vi "Read ADU Packet.vi"(8 "error in":errorcluster, 10 "protocol layer":refnum<class "Network Protocol.lvclass">, 11 "RTU transmission data unit in":refnum<class "RTU Data Unit.lvclass">) -> (0 "error out":errorcluster, 1 "modbus data unit":refnum<class "Modbus Data Unit (PDU).lvclass">, 2 "protocol layer out":refnum<class "Network Protocol.lvclass">, 3 "RTU transmission data unit out":refnum<class "RTU Data Unit.lvclass">, 5 "PDU Valid?":bool)   [LabVIEW 2020, in "SubVIs.lvlib" / "RTU Data Unit.lvclass"]
doc: "This uses the protocol layer to read a modbus packet off of the bus, wrapped in the RTU transmission data unit."
uses:
  <vilib>/Modbus/subvis/Transmission Data Unit (ADU)/RTU Data Unit/RTU Data Unit.lvclass
  C:/builds/penguin/iak/lvdsc/trunk/20.0/lv/vi.lib/Modbus/subvis/Transmission Data Unit (ADU)/Transmission Data Unit/Transmission Data Unit.lvclass
  C:/builds/penguin/iak/lvdsc/trunk/20.0/lv/vi.lib/Modbus/subvis/Transmission Data Unit (ADU)/Serial Data Unit/Serial Data Unit.lvclass
  <vilib>/Modbus/subvis/Modbus Data Unit (PDU)/Modbus Data Unit (PDU).lvclass
  <vilib>/Modbus/subvis/Protocol/Interfaces/Network Protocol/Network Protocol.lvclass
  <vilib>/Modbus/subvis/Protocol/Serial/Serial Slave/Serial Slave.lvclass
  <vilib>/Modbus/subvis/Protocol/Serial/Serial Master/Serial Master.lvclass
  <vilib>/Modbus/subvis/Protocol/Serial/Serial Master/Serial Master.lvclass/Serial Master.ctl
  <vilib>/Modbus/subvis/Protocol/Serial/Serial Slave/Serial Slave.lvclass/Serial Slave.ctl
  <vilib>/Modbus/subvis/Transmission Data Unit (ADU)/Transmission Data Unit/Transmission Data Unit.lvclass/Transmission Data Unit.ctl
  <vilib>/Modbus/subvis/Transmission Data Unit (ADU)/Serial Data Unit/Serial Data Unit.lvclass/Serial Data Unit.ctl
  <vilib>/Modbus/subvis/Modbus Data Unit (PDU)/Modbus Data Unit (PDU).lvclass/Modbus Data Unit (PDU).ctl
  <vilib>/ErrorRing/Error Ring.xnode
  <vilib>/Modbus/subvis/Transmission Data Unit (ADU)/Serial Data Unit/Serial Data Unit.lvclass
  <vilib>/Modbus/subvis/Transmission Data Unit (ADU)/Transmission Data Unit/Transmission Data Unit.lvclass
  <vilib>/Modbus/subvis/Protocol/Serial/Serial Shared Components/Serial Shared Components.lvlib
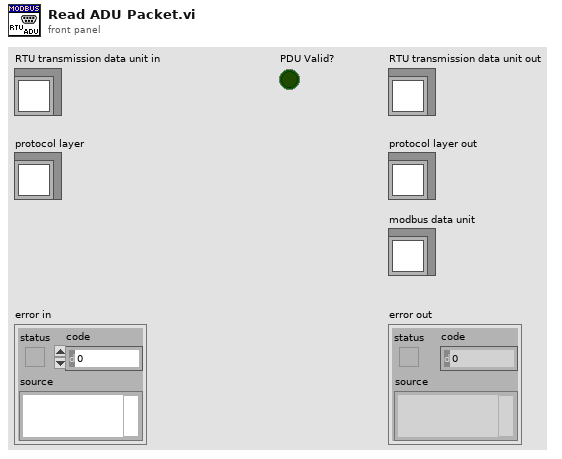
[diagram p1: front panel]
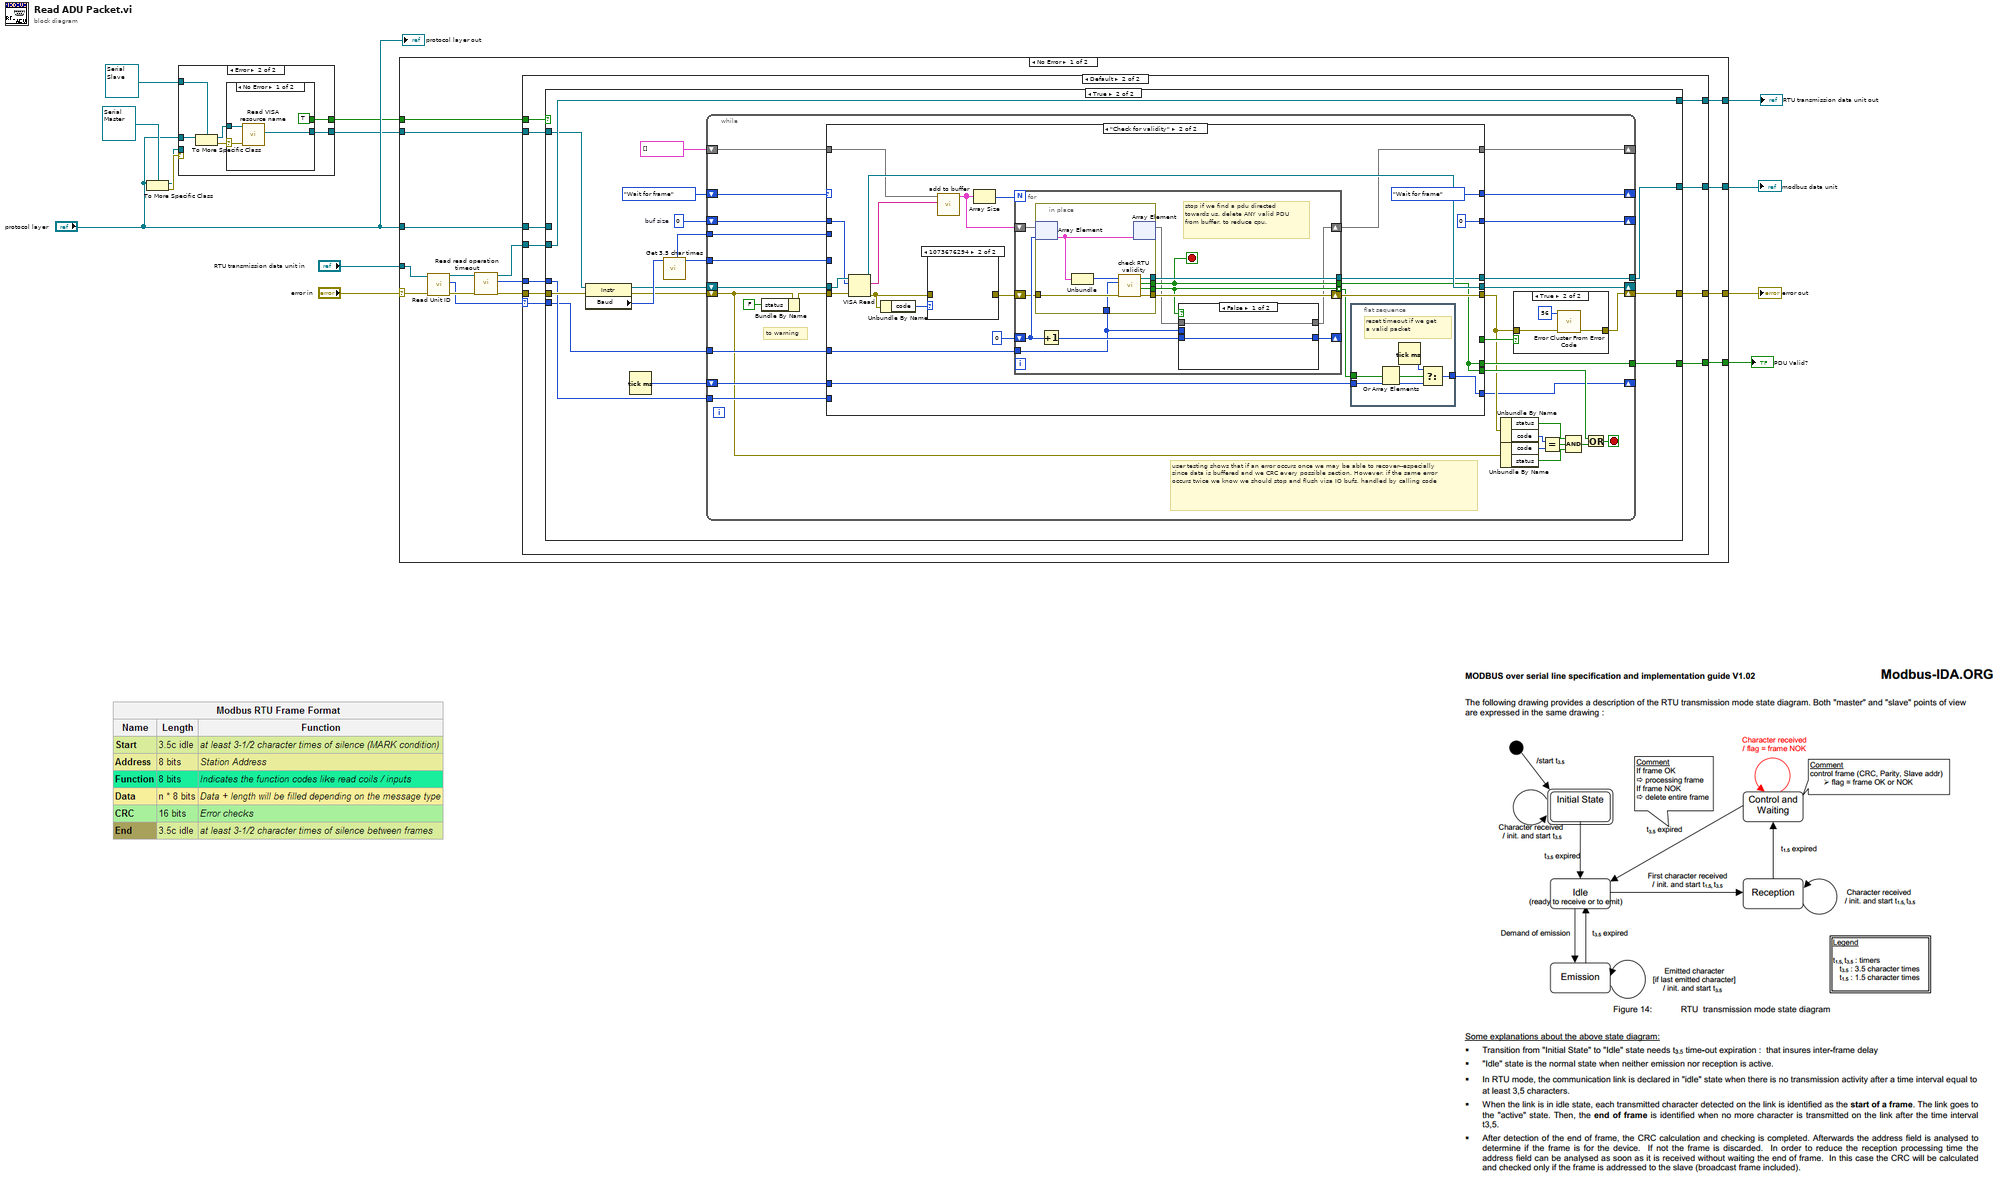
[diagram p0: block diagram]
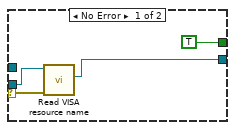
[diagram p2: hidden frame]
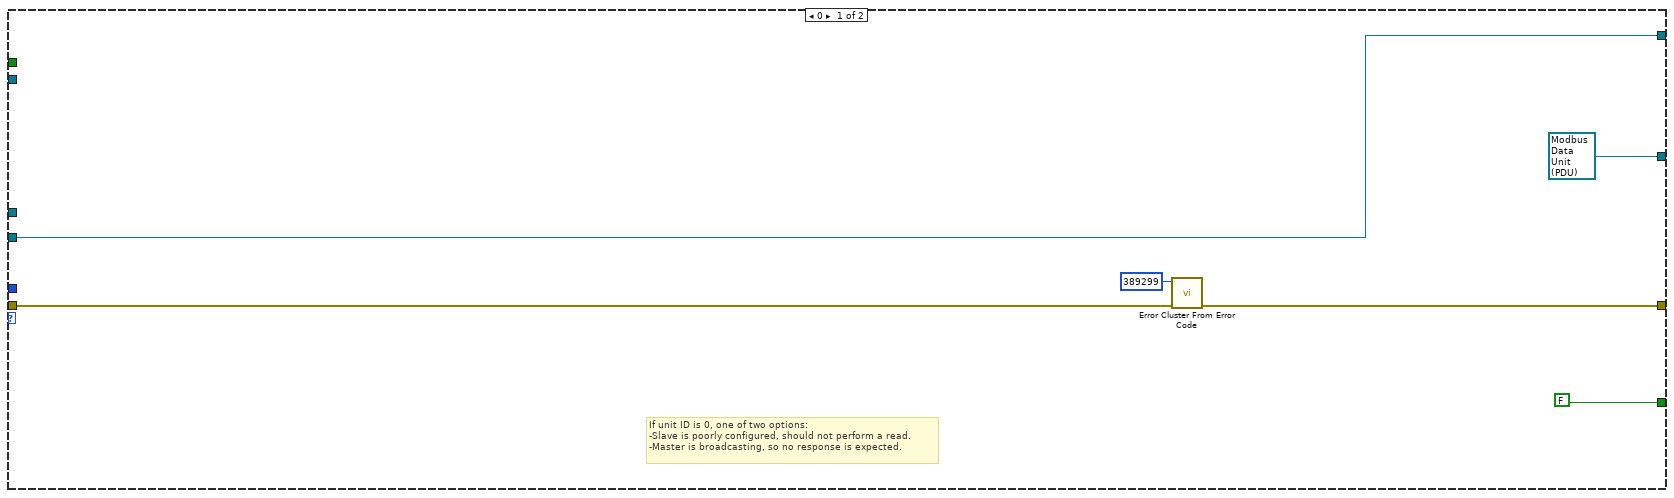
[diagram p4: hidden frame]
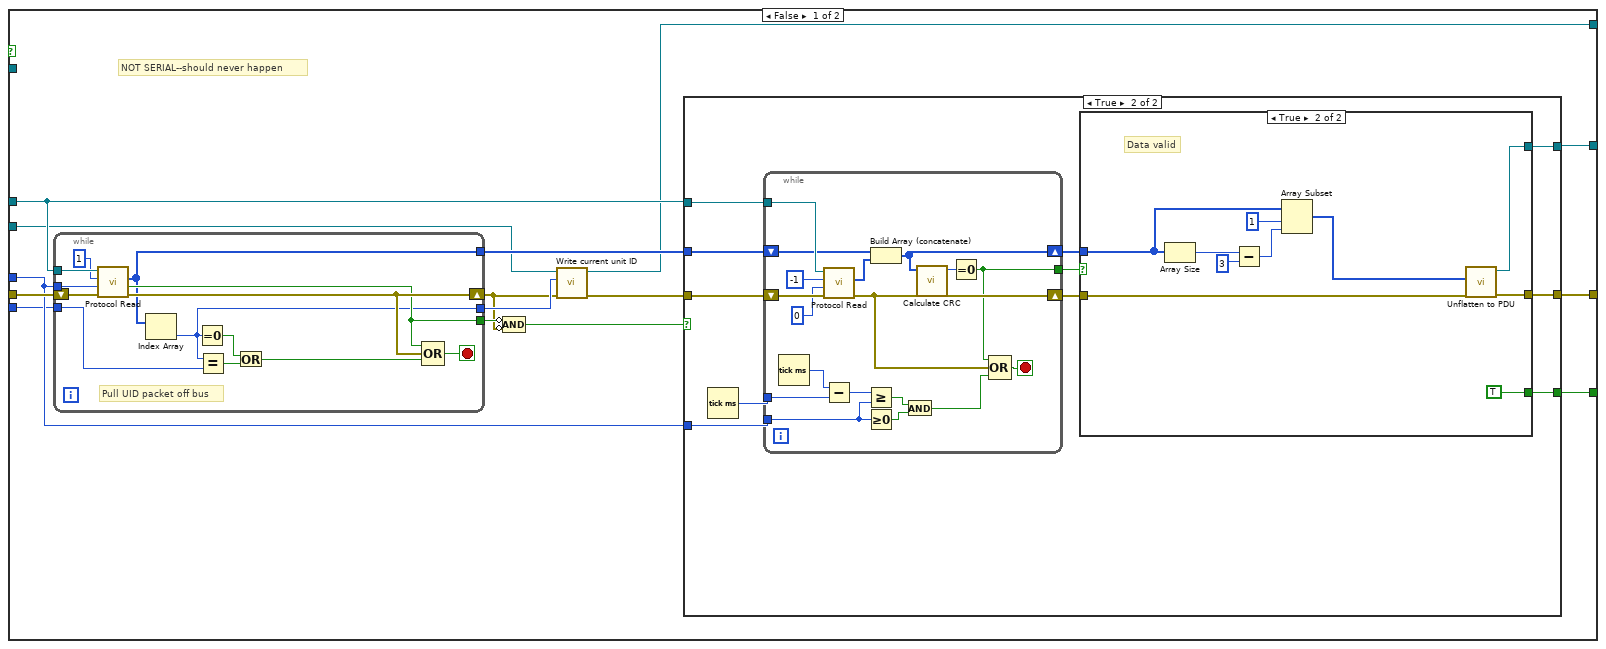
[diagram p5: hidden frame]
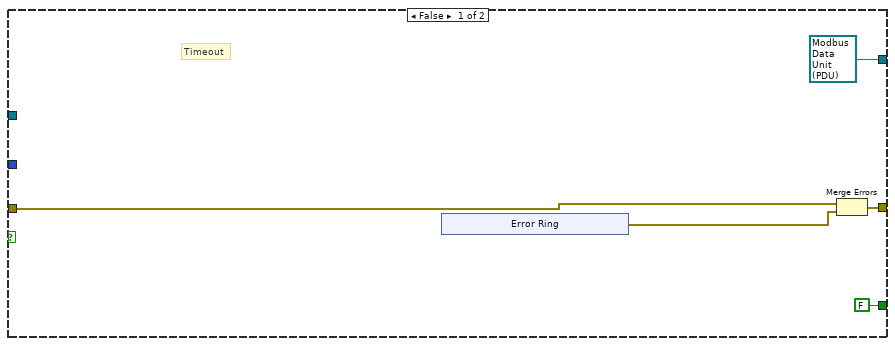
[diagram p6: hidden frame]
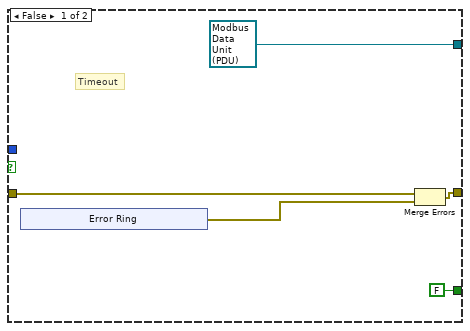
[diagram p7: hidden frame]
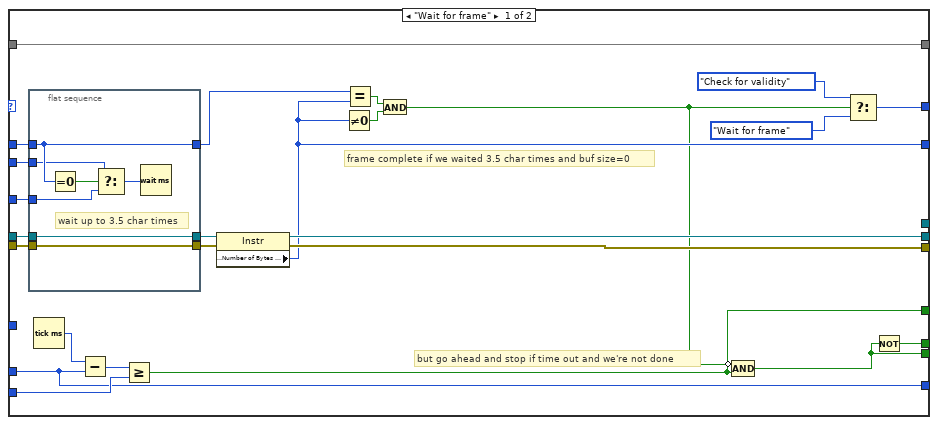
[diagram p9: hidden frame]
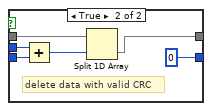
[diagram p11: hidden frame]
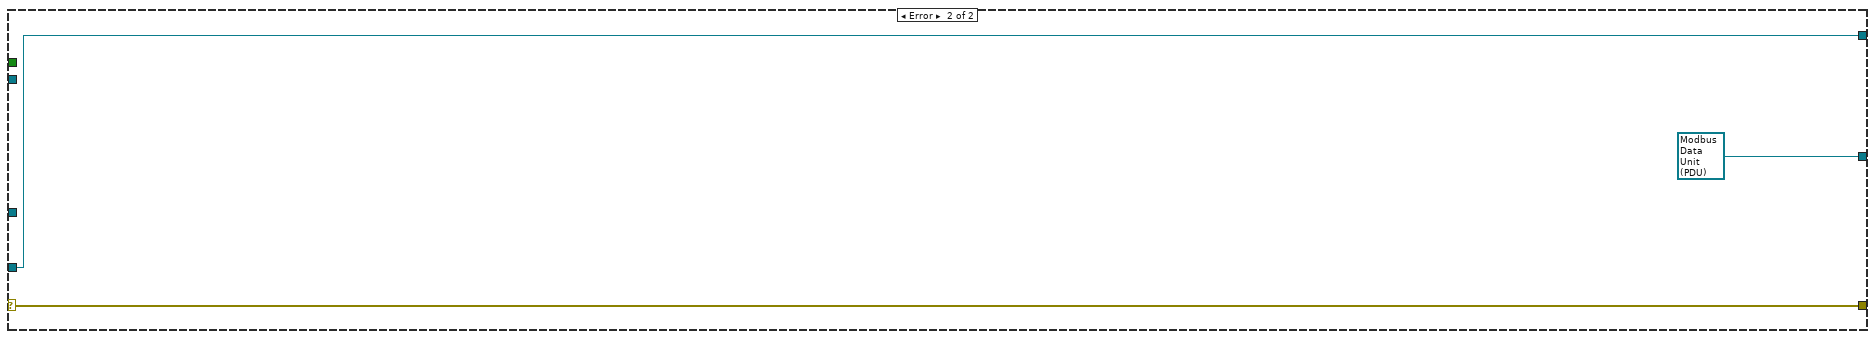
[diagram p12: hidden frame]
diagram:
  n1 = To More Specific Class(target class=refnum<class "Serial Master.lvclass"> refnum ("Serial Master"), reference="protocol layer") -> (specific class reference=w2:refnum<class "Serial Master.lvclass">, error out=w6:errorcluster)  [unwired: 1 in]
  n2 = case shown="Error" w6 {
    selector: w6 -> [w16 _]
    tunnel: "protocol layer" -> [_ w23]
    tunnel: [TRUE w21] -> w4
    tunnel: refnum<class "Serial Slave.lvclass"> refnum ("Serial Slave") -> [_ w20]
    tunnel: [w14 w18] -> w1
    tunnel: w2 -> [w15 _]
    frame No Error {
      n3 = call <vilib>:"Read VISA resource name.vi"("error in (no error)"=w16, "serial master in"=w15) -> ("VISA resource name"=w14:refnum<visa-resource-name>)  [unwired: 7 in, 2 out]
    }
    frame Error {
      n4 = To More Specific Class(target class=w20, reference=w23) -> (specific class reference=w19:refnum<class "Serial Slave.lvclass">, error out=w22:errorcluster)  [unwired: 1 in]
      n5 = case shown="No Error" w22 {
        selector: w22 -> [w26 _]
        tunnel: [TRUE _] -> w21
        tunnel: w19 -> [w25 _]
        tunnel: [w24 _] -> w18
        frame No Error {
          n6 = call <vilib>:"Read VISA resource name.vi"("error in (no error)"=w26, "serial slave in"=w25) -> ("VISA resource name"=w24:refnum<visa-resource-name>)  [unwired: 7 in, 2 out]
        }
        frame Error {
        }
      }
    }
  }
  n7 = case shown="No Error" "error in" {
    selector: "error in" -> [w35 w286]
    tunnel: [w42 w286] -> w12
    tunnel: "RTU transmission data unit in" -> [w36 w284]
    tunnel: "protocol layer" -> [w40 _]
    tunnel: [w41 refnum<class "Modbus Data Unit (PDU).lvclass"> refnum ("modbus data unit")] -> w11
    tunnel: [w39 w284] -> w9
    tunnel: [w30 _] -> w8
    tunnel: w4 -> [w29 _]
    tunnel: w1 -> [w28 _]
    frame No Error {
      n8 = call <vilib>:"Read Unit ID.vi"("error in"=w35, "transmission data unit in"=w36) -> ("error out"=w34:errorcluster, "unit ID"=w32:u8, "transmission data unit out"=w33:refnum<class "RTU Data Unit.lvclass">)  [unwired: 7 in]
      n9 = call <vilib>:"Read read operation timeout.vi"("error in (no error)"=w34, "transmission data unit in"=w33) -> ("error out"=w37:errorcluster, "read operation timeout"=w31:i32, "transmission data unit out"=w38:refnum<class "RTU Data Unit.lvclass">)  [unwired: 7 in]
      n10 = case shown="Default" w32 {
        selector: w32 -> [_ w54]
        tunnel: w37 -> [w48 w59]
        tunnel: [w44 w58] -> w42
        tunnel: [refnum<class "Modbus Data Unit (PDU).lvclass"> refnum ("modbus data unit out") w57] -> w41
        tunnel: w40 -> [_ w56]
        tunnel: w31 -> [_ w55]
        tunnel: w38 -> [w47 w52]
        tunnel: [w47 w53] -> w39
        tunnel: [FALSE w51] -> w30
        tunnel: w29 -> [_ w50]
        tunnel: w28 -> [_ w49]
        frame 0 {
          # "If unit ID is 0, one of two options:\n-Slave is poorly configured, should not perform a read.\n-Master is broadcasting, so no response is expected."
          n11 = call <vilib>:"Error Cluster From Error Code.vi"("error in (no error)"=w48, "error code (0)"=389299) -> ("error out"=w44:errorcluster)  [unwired: 7 in]
        }
        frame Default {
          n12 = case shown="True" w50 {
            tunnel: w59 -> [w74 w159]
            tunnel: [w71 w156] -> w58
            tunnel: [w70 w147] -> w57
            tunnel: w56 -> [w69 _]
            tunnel: w55 -> [w67 w151]
            tunnel: w54 -> [w66 w148]
            tunnel: [w65 w161] -> w53
            tunnel: w52 -> [w63 w161]
            tunnel: [w60 w149] -> w51
            tunnel: w49 -> [_ w158]
            frame False {
              # "NOT SERIAL--should never happen"
              n13 = while {
                shift-right: [w141] -> w61
                shift-left: w74 -> [w144]
                tunnel: w67 -> [w139]
                tunnel: w66 -> [w135]
                tunnel: [w134] -> w73
                tunnel: [w133] -> w68
                tunnel: w69 -> [w143]
                tunnel: [w132] -> w62
                stop <- w142 stop-if-true
                # "Pull UID packet off bus"
                n14 = call-dynamic "Protocol Read.vi"("error in (no error)"=w144, "timeout"=w139, "bytes to read"=1, "protocol layer in"=w143) -> ("error out"=w141:errorcluster, "timed out?"=w134:bool, "data"=w133:u8[])  [unwired: 4 in, 1 out]
                n15 = Index Array(array=w133) -> (element=w132:u8)  [unwired: 1 in]
                n16 = Equal To 0?(x=w132) -> (x = 0?=w136:bool)
                n17 = Equal?(x=w132, y=w135) -> (x = y?=w138:bool)
                n18 = Or(x=w136, y=w138) -> (x .or. y?=w137:bool)
                n19 = Compound Arithmetic op=OR(w134, w141, w137) -> (w142:bool)
              }
              n20 = Compound Arithmetic op=AND(invert w73, invert w61) -> (w72:bool)
              n21 = call <vilib>:"Write current unit ID.vi"("error in (no error)"=w61, "request unit ID"=w62, "serial data unit in"=w63) -> ("error out"=w64:errorcluster, "serial data unit out"=w65:refnum<class "RTU Data Unit.lvclass">)  [unwired: 7 in]
              n22 = case shown="True" w72 {
                tunnel: w64 -> [w77 w94]
                tunnel: [w78 w86] -> w71
                tunnel: [refnum<class "Modbus Data Unit (PDU).lvclass"> refnum ("modbus data unit out") w87] -> w70
                tunnel: w69 -> [_ w90]
                tunnel: w68 -> [_ w91]
                tunnel: w67 -> [_ w92]
                tunnel: [FALSE w84] -> w60
                frame False {
                  # "Timeout"
                  n23 = xnode "Error Ring"() -> ("error out"=w79:errorcluster)
                  n24 = Merge Errors(w77, w79) -> (w78:errorcluster)
                }
                frame True {
                  n25 = Tick Count (ms)() -> (millisecond timer value=w93:u32)
                  n26 = while {
                    shift-right: [w117] -> w88
                    shift-left: w94 -> [w123]
                    tunnel: w93 -> [w131]
                    tunnel: w92 -> [w128]
                    shift-right: [w115] -> w85
                    shift-left: w91 -> [w119]
                    tunnel: w90 -> [w122]
                    tunnel: [w114] -> w89
                    stop <- w125 stop-if-true
                    n27 = Tick Count (ms)() -> (millisecond timer value=w130:u32)
                    n28 = call-dynamic "Protocol Read.vi"("error in (no error)"=w123, "timeout"=0, "bytes to read"=-1, "protocol layer in"=w122) -> ("error out"=w117:errorcluster, "data"=w118:u8[])  [unwired: 4 in, 2 out]
                    n29 = Subtract(x=w130, y=w131) -> (x-y=w129:u32)
                    n30 = Greater Or Equal?(x=w129, y=w128) -> (x >= y?=w126:bool)
                    n31 = Greater Or Equal To 0?(x=w128) -> (x >= 0?=w127:bool)
                    n32 = Build Array (concatenate)(w119, w118) -> (w115:u8[])
                    n33 = And(x=w126, y=w127) -> (x .and. y?=w124:bool)
                    n34 = call <vilib>:"Calculate CRC.vi"("data"=w115) -> ("CRC-16"=w116:u16)  [unwired: 10 in]
                    n35 = Equal To 0?(x=w116) -> (x = 0?=w114:bool)
                    n36 = Compound Arithmetic op=OR(w114, w117, w124) -> (w125:bool)
                  }
                  n37 = case shown="True" w89 {
                    tunnel: w88 -> [w97 w111]
                    tunnel: [refnum<class "Modbus Data Unit (PDU).lvclass"> refnum ("modbus data unit") w112] -> w87
                    tunnel: [w96 w113] -> w86
                    tunnel: w85 -> [_ w105]
                    tunnel: [FALSE TRUE] -> w84
                    frame False {
                      # "Timeout"
                      n38 = xnode "Error Ring"() -> ("error out"=w98:errorcluster)
                      n39 = Merge Errors(w97, w98) -> (w96:errorcluster)
                    }
                    frame True {
                      # "Data valid"
                      n40 = Array Size(array=w105) -> (size(s)=w109:i32)
                      n41 = Subtract(x=w109, y=3) -> (x-y=w107:i32)
                      n42 = Array Subset(array=w105, index=1, length=w107) -> (w106:u8[])
                      n43 = call <vilib>:"Unflatten to PDU.vi"("error in (no error)"=w111, "Modbus data unit data"=w106) -> ("error out"=w113:errorcluster, "Modbus data unit out"=w112:refnum<class "Modbus Data Unit (PDU).lvclass">)  [unwired: 8 in]
                    }
                  }
                }
              }
            }
            frame True {
              w153 = u32 0  # buf size
              n44 = property class="Instr"(reference=w158, error in=w159) -> (reference out=w155:refnum<visa-resource-name>, error out=w157:errorcluster, "Baud"=w160:u32)
              n45 = Tick Count (ms)() -> (millisecond timer value=w152:u32)
              n46 = call <vilib>:"Get 3.5 char times.vi"("baud rate"=w160) -> ("wait time (ms)"=w150:u32, "default wait (ms)"=w145:u32)  [unwired: 9 in]
              n47 = while {
                shift-right: [w177] -> w156
                shift-left: w157 -> [w173]
                shift-right: [w183] -> _
                shift-left: w155 -> [w190]
                shift-right: [w182] -> _
                shift-left: enum16{"Wait for frame", "Check for validity"}."Wait for frame" ("Serial Acquisition States") -> [w191]
                shift-right: [w185] -> _
                shift-left: w153 -> [w187]
                tunnel: w151 -> [w188]
                tunnel: w150 -> [w186]
                tunnel: [w181] -> w149
                tunnel: w148 -> [w180]
                tunnel: [w179] -> w147
                shift-right: [w165] -> _
                shift-left: cluster{"data":u8[], "packets contained":i32}[] [] -> [w164]
                shift-right: [w163] -> _
                shift-left: w152 -> [w189]
                tunnel: w145 -> [w162]
                stop <- w167 stop-if-true
                # "user testing shows that if an error occurs once we may be able to recover--especially since data is buffered and we CRC every possible section. However, if the same error occurs twice we know we should stop and flush visa IO bufs, handled by calling code"
                # "to warning"
                n48 = Bundle By Name(cluster=w173, "status"=FALSE) -> (w176:errorcluster)
                n49 = case shown="\"Check for validity\"" w191 {
                  tunnel: w190 -> [w216 w248]
                  tunnel: w176 -> [w215 w249]
                  tunnel: w189 -> [w197 w233]
                  tunnel: w188 -> [w218 _]
                  tunnel: w187 -> [w213 w247]
                  tunnel: w186 -> [w212 _]
                  tunnel: [w203 u32 0 ("Bytes at Port")] -> w185
                  tunnel: [w200 w234] -> w184
                  tunnel: [w208 w239] -> w174
                  tunnel: [w207 w245] -> w183
                  tunnel: [w204 enum16{"Wait for frame", "Check for validity"}."Wait for frame" ("Serial Acquisition States")] -> w182
                  tunnel: [w201 w234] -> w181
                  tunnel: w180 -> [_ w236]
                  tunnel: [_ w235] -> w179
                  tunnel: [w199 _] -> w178
                  tunnel: [w198 w237] -> w165
                  tunnel: w164 -> [w198 w243]
                  tunnel: [w197 w232] -> w163
                  tunnel: w162 -> [w196 _]
                  frame "Wait for frame" {
                    # "but go ahead and stop if time out and we're not done"
                    # "frame complete if we waited 3.5 char times and buf size=0"
                    n50 = flat-sequence {
                      tunnel: [w227] -> w217
                      tunnel: w216 -> [w227]
                      tunnel: w215 -> [w226]
                      tunnel: [w226] -> w214
                      tunnel: w213 -> [w225]
                      tunnel: [w225] -> w209
                      tunnel: w212 -> [w223]
                      tunnel: w196 -> [w221]
                      frame #0 {
                        # "wait up to 3.5 char times"
                        n51 = Equal To 0?(x=w225) -> (x = 0?=w224:bool)
                        n52 = Select(t=w221, s=w224, f=w223) -> (s? t:f=w222:u32)
                        n53 = Wait (ms)(milliseconds to wait=w222) -> ()  [unwired: 1 out]
                      }
                    }
                    n54 = Tick Count (ms)() -> (millisecond timer value=w220:u32)
                    n55 = Subtract(x=w220, y=w197) -> (x-y=w219:u32)
                    n56 = Greater Or Equal?(x=w219, y=w218) -> (x >= y?=w199:bool)
                    n57 = property class="Instr"(reference=w217, error in=w214) -> (reference out=w207:refnum<visa-resource-name>, error out=w208:errorcluster, "Serial Settings:Number of Bytes at Serial Port"=w203:u32)
                    n58 = Not Equal To 0?(x=w203) -> (x != 0?=w211:bool)
                    n59 = Equal?(x=w209, y=w203) -> (x = y?=w210:bool)
                    n60 = And(x=w210, y=w211) -> (x .and. y?=w202:bool)
                    n61 = Compound Arithmetic op=AND(invert w202, w199) -> (w200:bool)
                    n62 = Select(t=enum16{"Wait for frame", "Check for validity"}."Check for validity" ("Serial Acquisition States"), s=w202, f=enum16{"Wait for frame", "Check for validity"}."Wait for frame" ("Serial Acquisition States")) -> (s? t:f=w204:enum16{"Wait for frame", "Check for validity"})
                    n63 = Not(x=w200) -> (.not. x?=w201:bool)
                  }
                  frame "Check for validity" {
                    n64 = VISA Read(VISA resource name=w248, byte count=w247, error in (no error)=w249) -> (VISA resource name out=w245:refnum<visa-resource-name>, read buffer=w242:string, error out=w229:errorcluster)  [unwired: 1 out]
                    n65 = Unbundle By Name(w229) -> ("code"=w230:i32)
                    n66 = case shown="1073676294" w230 {
                      tunnel: [w250 _] -> w228
                      tunnel: w229 -> [w250 _]
                      frame Default {
                      }
                      frame 1073676294 {
                      }
                    }
                    n67 = call <vilib>:"add to buffer.vi"("read data"=w242, "buffer in"=w243) -> ("buffer out"=w240:cluster{"data":u8[], "packets contained":i32}[])  [unwired: 9 in]
                    n68 = Array Size(array=w240) -> (size(s)=w241:i32)
                    n69 = for {
                      N: w241 -> [_]
                      shift-right: [w257] -> w237
                      shift-left: w240 -> [w267]
                      shift-right: [w264] -> w239
                      shift-left: w228 -> [w265]
                      tunnel: w236 -> [w256]
                      tunnel: [w263] -> w235
                      tunnel: [w262] -> w234
                      tunnel: [w261] -> w231 mode=indexing
                      shift-right: [w260] -> _
                      shift-left: 0 -> [w266]
                      stop <- w262 stop-if-true
                      # "stop if we find a pdu directed towards us. delete ANY valid PDU from buffer, to reduce cpu."
                      n70 = in-place {
                        in-place-border: w265 -> [w283]
                        in-place-border: [w280] -> w263
                        in-place-border: [w279] -> w262
                        in-place-border: [w278] -> w261
                        in-place-border: [w277] -> w264
                        in-place-border: w256 -> [w276]
                        n71 = in-place-array #1(w267, w266) -> (w281:cluster{"data":u8[], "packets contained":i32})
                        n72 = Unbundle(w281) -> ("data"=w282:u8[])  [unwired: 1 out]
                        n73 = call <vilib>:"check RTU validity.vi"("error in (no error)"=w283, "unit ID"=w276, "unsigned byte array"=w282) -> ("error out"=w277:errorcluster, "valid packet"=w278:bool, "valid PDU"=w279:bool, "Modbus data unit out"=w280:refnum<class "Modbus Data Unit (PDU).lvclass">)  [unwired: 5 in]
                        n74 = in-place-array #1(w281) -> (w258:cluster{"data":u8[], "packets contained":i32}[])  [unwired: 1 out]
                      }
                      n75 = Increment(x=w266) -> (x+1=w259:i32)
                      n76 = case shown="False" w261 {
                        tunnel: [w269 0] -> w260
                        tunnel: w259 -> [w269 w274]
                        tunnel: w258 -> [w268 w272]
                        tunnel: [w268 w270] -> w257
                        tunnel: w256 -> [_ w273]
                        frame False {
                        }
                        frame True {
                          # "delete data with valid CRC"
                          n77 = Add(x=w273, y=w274) -> (x+y=w271:i32)
                          n78 = Split 1D Array(array=w272, index=w271) -> (second subarray=w270:cluster{"data":u8[], "packets contained":i32}[])  [unwired: 1 out]
                        }
                      }
                    }
                    n79 = flat-sequence {
                      tunnel: w233 -> [w255]
                      tunnel: [w254] -> w232
                      tunnel: w231 -> [w251]
                      frame #0 {
                        # "reset timeout if we get\na valid packet"
                        n80 = Or Array Elements(Boolean array=w251) -> (logical OR=w252:bool)
                        n81 = Tick Count (ms)() -> (millisecond timer value=w253:u32)
                        n82 = Select(t=w253, s=w252, f=w255) -> (s? t:f=w254:u32)
                      }
                    }
                  }
                }
                n83 = Unbundle By Name(w174) -> ("status"=w170:bool, "code"=w171:i32)
                n84 = Unbundle By Name(w173) -> ("code"=w172:i32, "status"=w168:bool)
                n85 = case shown="True" w178 {
                  tunnel: w174 -> [w192 w195]
                  tunnel: [w192 w194] -> w177
                  frame False {
                  }
                  frame True {
                    n86 = call <vilib>:"Error Cluster From Error Code.vi"("error in (no error)"=w195, "error code (0)"=56) -> ("error out"=w194:errorcluster)  [unwired: 7 in]
                  }
                }
                n87 = Equal?(x=w171, y=w172) -> (x = y?=w169:bool)
                n88 = Compound Arithmetic op=AND(w170, w169, w168) -> (w166:bool)
                n89 = Or(x=w184, y=w166) -> (x .or. y?=w167:bool)
              }
            }
          }
        }
      }
    }
    frame Error {
    }
  }
  "RTU transmission data unit out" <- w9
  "modbus data unit" <- w11
  "error out" <- w12
  "PDU Valid?" <- w8
  "protocol layer out" <- "protocol layer"
